vi "4Pi Capture Write ini File.vi"(7 "type":T1, 8 "property name":string, 9 "section name":string, 10 "Variant":variant, 11 "Refnum in":T2) -> (0 "error out":errorcluster, 3 "Refnum out":T2)   [LabVIEW 2021]
uses:
  <vilib>/Utility/config.llb/Config Data RefNum.ctl
  <vilib>/Utility/Data Type/Type Definitions/Data Type.ctl
  <vilib>/Utility/config.llb/Write Key (Double).vi
  <vilib>/Utility/config.llb/Write Key (I32).vi
  <vilib>/Utility/config.llb/Write Key (U32).vi
  <vilib>/Utility/config.llb/Write Key (Boolean).vi
  <vilib>/Utility/config.llb/Write Key (String).vi
  <vilib>/Utility/config.llb/Write Key (Path).vi
  <vilib>/Utility/config.llb/NI_LVConfig.lvlib
  <vilib>/Utility/Data Type/NI_Data Type.lvlib
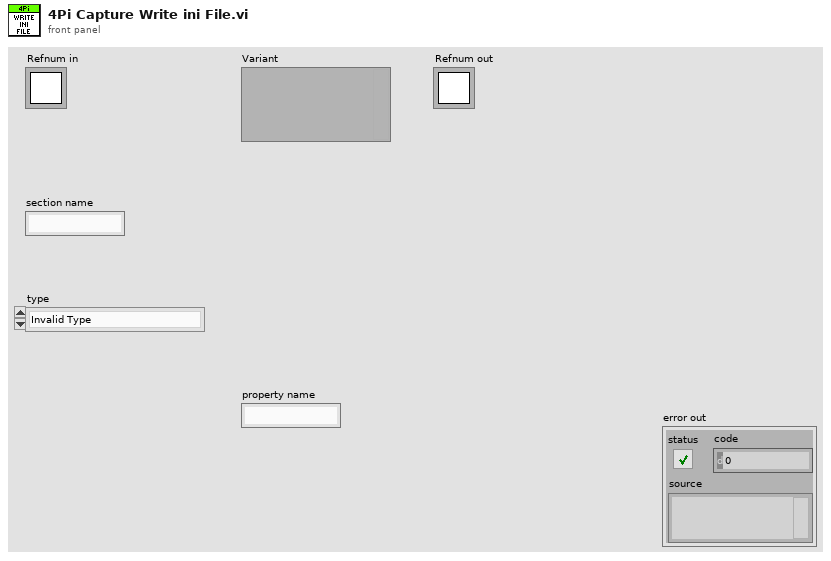
[diagram p1: front panel]
types:
  T1 = typedef "NI_Data Type.lvlib/Data Type.ctl" = enum8{"Invalid Type", "Void", "I8", "I16", "I32", "I64", "U8", "U16", "U32", "U64", "Single Float", "Double Float", "Extended Float", "Single Complex", "Double Complex", "Extended Complex", "Enum U8", "Enum U16", "Enum U32", "Enum U64", "Single Float With Unit", "Double Float With Unit", "Extended Float With Unit", "Single Complex with Unit", "Double Complex with Unit", "Extended Complex with Unit", "Boolean", "String", "Path", "Picture", "Tag", "Array", "Cluster", "Variant", "LV Variant", "Waveform", "Timestamp", "Digital Waveform", "Digital Data", "ExpressData", "Refnum", "External Data", "VI", "Poly VI", "LabVIEW Class Instance", "Fixed Point", "Set Collection", "Map Collection"}
  T2 = typedef "NI_LVConfig.lvlib/Config Data RefNum.ctl" = refnum<k1>
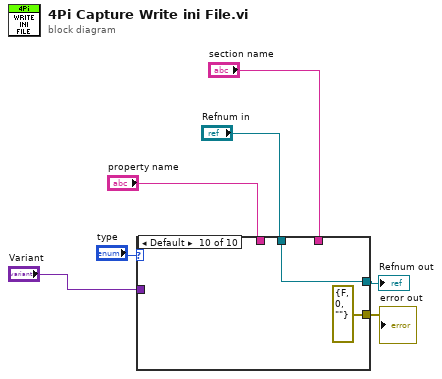
[diagram p0: block diagram]
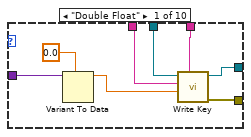
[diagram p2: hidden frame]
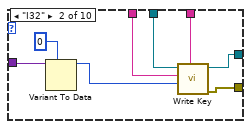
[diagram p3: hidden frame]
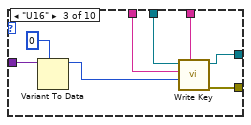
[diagram p4: hidden frame]
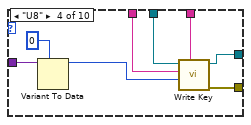
[diagram p5: hidden frame]
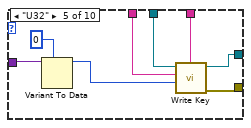
[diagram p6: hidden frame]
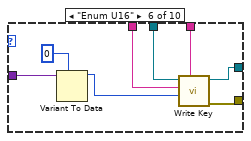
[diagram p7: hidden frame]
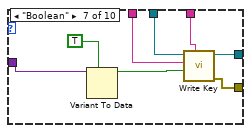
[diagram p8: hidden frame]
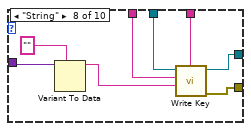
[diagram p9: hidden frame]
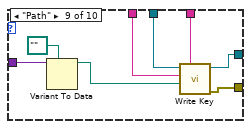
[diagram p10: hidden frame]
diagram:
  n1 = case shown="Default" "type" {
    tunnel: "Variant" -> [w15 w23 w31 w39 w47 w49 w63 w71 w73 _]
    tunnel: "Refnum in" -> [w9 w20 w28 w36 w44 w54 w61 w68 w77 w81]
    tunnel: [w10 w17 w25 w34 w41 w52 w60 w65 w74 w81] -> w7
    tunnel: "section name" -> [w11 w21 w29 w37 w45 w55 w59 w69 w78 _]
    tunnel: "property name" -> [w13 w19 w27 w35 w42 w53 w57 w67 w76 _]
    tunnel: [w8 w16 w24 w32 w40 w48 w56 w64 w72 errorcluster {"status"=FALSE, "code"=0, "source"=""} ("error out")] -> w1
    frame "Double Float" {
      n2 = Variant To Data(type=0.0, Variant=w15) -> (data=w12:dbl)  [unwired: 1 in, 1 out]
      n3 = call-poly <vilib>:"Write Key.vi"("section"=w11, "value"=w12, "key"=w13, "refnum"=w9) -> ("error out"=w8:errorcluster, "refnum out"=w10:T2)  [unwired: 5 in, 1 out]
    }
    frame "I32" {
      n4 = Variant To Data(type=0, Variant=w23) -> (data=w18:i32)  [unwired: 1 in, 1 out]
      n5 = call-poly <vilib>:"Write Key.vi"("section"=w21, "value"=w18, "key"=w19, "refnum"=w20) -> ("error out"=w16:errorcluster, "refnum out"=w17:T2)  [unwired: 5 in, 1 out]
    }
    frame "U16" {
      n6 = Variant To Data(type=u16 0, Variant=w31) -> (data=w26:u16)  [unwired: 1 in, 1 out]
      n7 = call-poly <vilib>:"Write Key.vi"("section"=w29, "value"=w26, "key"=w27, "refnum"=w28) -> ("error out"=w24:errorcluster, "refnum out"=w25:T2)  [unwired: 5 in, 1 out]
    }
    frame "U8" {
      n8 = Variant To Data(type=u8 0, Variant=w39) -> (data=w33:u8)  [unwired: 1 in, 1 out]
      n9 = call-poly <vilib>:"Write Key.vi"("section"=w37, "value"=w33, "key"=w35, "refnum"=w36) -> ("error out"=w32:errorcluster, "refnum out"=w34:T2)  [unwired: 5 in, 1 out]
    }
    frame "U32" {
      n10 = Variant To Data(type=u32 0, Variant=w47) -> (data=w43:u32)  [unwired: 1 in, 1 out]
      n11 = call-poly <vilib>:"Write Key.vi"("section"=w45, "value"=w43, "key"=w42, "refnum"=w44) -> ("error out"=w40:errorcluster, "refnum out"=w41:T2)  [unwired: 5 in, 1 out]
    }
    frame "Enum U16" {
      n12 = Variant To Data(type=0, Variant=w49) -> (data=w50:i32)  [unwired: 1 in, 1 out]
      n13 = call-poly <vilib>:"Write Key.vi"("section"=w55, "value"=w50, "key"=w53, "refnum"=w54) -> ("error out"=w48:errorcluster, "refnum out"=w52:T2)  [unwired: 5 in, 1 out]
    }
    frame "Boolean" {
      n14 = Variant To Data(type=TRUE, Variant=w63) -> (data=w58:bool)  [unwired: 1 in, 1 out]
      n15 = call-poly <vilib>:"Write Key.vi"("section"=w59, "value"=w58, "key"=w57, "refnum"=w61) -> ("error out"=w56:errorcluster, "refnum out"=w60:T2)  [unwired: 5 in, 1 out]
    }
    frame "String" {
      n16 = Variant To Data(type="", Variant=w71) -> (data=w66:string)  [unwired: 1 in, 1 out]
      n17 = call-poly <vilib>:"Write Key.vi"("section"=w69, "value"=w66, "key"=w67, "refnum"=w68) -> ("error out"=w64:errorcluster, "refnum out"=w65:T2)  [unwired: 5 in, 1 out]
    }
    frame "Path" {
      n18 = Variant To Data(type=path "", Variant=w73) -> (data=w75:path)  [unwired: 1 in, 1 out]
      n19 = call-poly <vilib>:"Write Key.vi"("section"=w78, "value"=w75, "key"=w76, "refnum"=w77) -> ("error out"=w72:errorcluster, "refnum out"=w74:T2)  [unwired: 5 in, 1 out]
    }
    frame Default {
    }
  }
  "Refnum out" <- w7
  "error out" <- w1
